vi "DriveWaitForButton.vi"() -> (0 "Error Out":errorcluster, 1 "Increment":bool)   [LabVIEW 2020]
doc: "This VI pauses the drive sequencer until the driver presses the \"advance system check\" button on the joystick, the joystick will rumble while waiting for the button.\n\nParameters:\nNone"
uses:
  GlobalDriverStationCommands.vi
  GlobalDriverStationData.vi
  GlobalAutonomous.vi
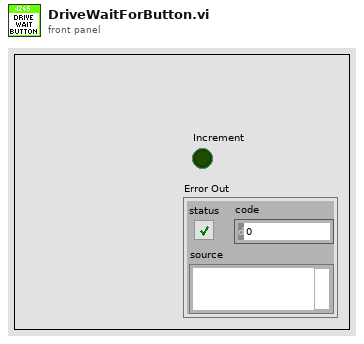
[diagram p1: front panel]
types:
  T1 = enum16{"Center", "North", "NorthWest", "West", "SouthWest", "South", "SouthEast", "East", "NorthEast"}
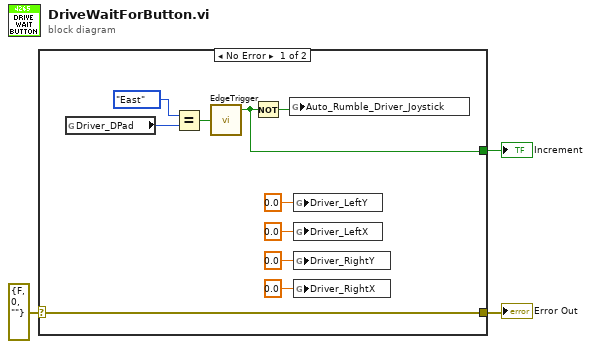
[diagram p0: block diagram]
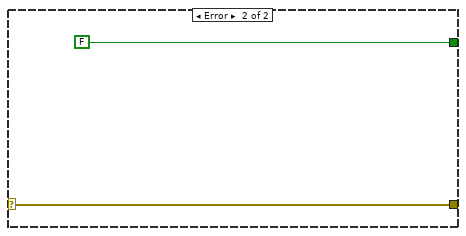
[diagram p2: hidden frame]
diagram:
  n1 = case shown="No Error" errorcluster {"status"=FALSE, "code"=0, "source"=""} ("error IO") {
    selector: errorcluster {"status"=FALSE, "code"=0, "source"=""} ("error IO") -> [w9 w15]
    tunnel: [w4 FALSE] -> w3
    tunnel: [w9 w15] -> w2
    frame No Error {
      n2 = global read "GlobalDriverStationData.vi" "Driver_DPad"() -> (w8:T1)
      n3 = Equal?(x=T1."East" ("Driver_DPad"), y=w8) -> (x = y?=w6:bool)
      n4 = call "EdgeTrigger.vi"("Input Signal"=w6) -> ("Rising Edge Trigger"=w4:bool)  [unwired: 2 out]
      n5 = Not(x=w4) -> (.not. x?=w7:bool)
      n6 = global write "GlobalAutonomous.vi" "Auto_Rumble_Driver_Joystick"(w7) -> ()
      n7 = global write "GlobalDriverStationCommands.vi" "Driver_LeftY"(0.0 ("Driver_LeftY")) -> ()
      n8 = global write "GlobalDriverStationCommands.vi" "Driver_LeftX"(0.0 ("Driver_RightX")) -> ()
      n9 = global write "GlobalDriverStationCommands.vi" "Driver_RightY"(0.0 ("Driver_RightX")) -> ()
      n10 = global write "GlobalDriverStationCommands.vi" "Driver_RightX"(0.0 ("Driver_RightX")) -> ()
    }
    frame Error {
    }
  }
  "Increment" <- w3
  "Error Out" <- w2
